vi "Partcalpm Control&FB.vi"(10 "Enum":T1(ring)) -> (2 "Part UnClamp Feedback":bool, 3 "Part Clamp Feedback":bool)   [LabVIEW 2015]
uses:
  Galobal variable_TI.vi
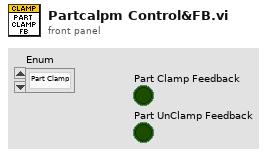
[diagram p1: front panel]
types:
  T1 = enum16{"Part Clamp", "Part Unclamp", "Part Clamp Input Check", "Part Unclamp Input Check"}
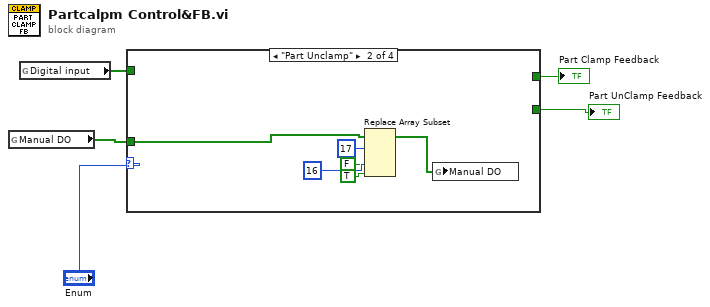
[diagram p0: block diagram]
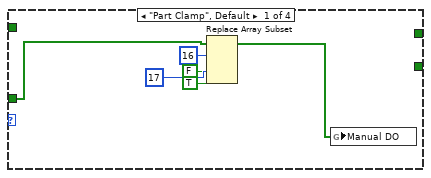
[diagram p2: hidden frame]
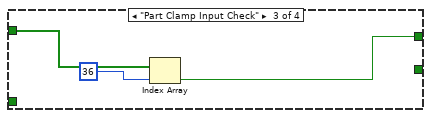
[diagram p3: hidden frame]
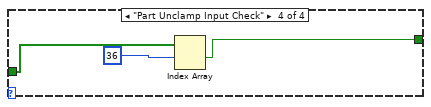
[diagram p4: hidden frame]
diagram:
  n1 = global read "Galobal variable_TI.vi" "Manual DO"() -> (w1:bool[])
  n2 = global read "Galobal variable_TI.vi" "Digital input"() -> (w4:bool[])
  n3 = case shown="\"Part Unclamp\"" "Enum" {
    tunnel: w1 -> [w9 w14 _ w21]
    tunnel: w4 -> [_ _ w20 _]
    tunnel: [_ _ w18 _] -> w3
    tunnel: [_ _ _ w22] -> w2
    frame "Part Clamp", Default {
      n4 = Replace Array Subset(array=w9, new element #1=FALSE ("new element/subarray"), index #1=16 ("index"), new element #2=TRUE ("new element/subarray"), index #2=17 ("index")) -> (w8:bool[])
      n5 = global write "Galobal variable_TI.vi" "Manual DO"(w8) -> ()
    }
    frame "Part Unclamp" {
      n6 = Replace Array Subset(array=w14, new element #1=FALSE ("new element/subarray"), index #1=17 ("index"), new element #2=TRUE ("new element/subarray"), index #2=16 ("index")) -> (w13:bool[])
      n7 = global write "Galobal variable_TI.vi" "Manual DO"(w13) -> ()
    }
    frame "Part Clamp Input Check" {
      n8 = Index Array(array=w20, index=36) -> (element=w18:bool)
    }
    frame "Part Unclamp Input Check" {
      n9 = Index Array(array=w21, index #1=36 ("index")) -> (element #1=w22:bool)  [unwired: 1 in, 1 out]
    }
  }
  "Part Clamp Feedback" <- w3
  "Part UnClamp Feedback" <- w2
